vi "Data_Process_Mass.vi"(7 "Frequency Spectrum":cluster{sgl[], sgl[]}, 8 "error in":errorcluster, 9 "Mag. Frequency (kHz)":dbl format="%.5g", 10 "Cycl. Frequency (kHz)":dbl format="%.5g", 11 "Reference mass (u)":dbl format="%.5g") -> (0 "error out":errorcluster caption="sortie d'erreur", 3 "Mass Spectrum":cluster{"mass":sgl[], sgl[]})   [LabVIEW 2020]
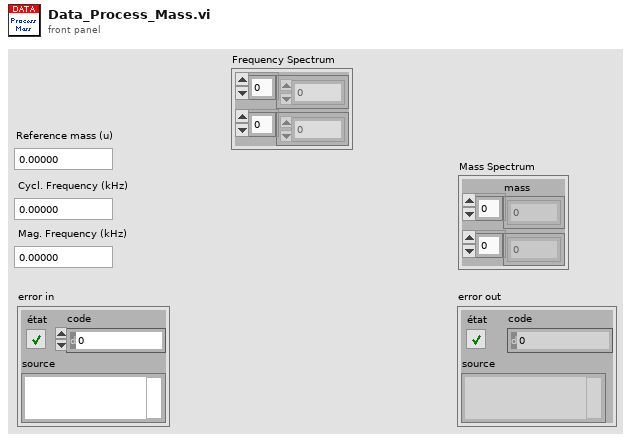
[diagram p1: front panel]
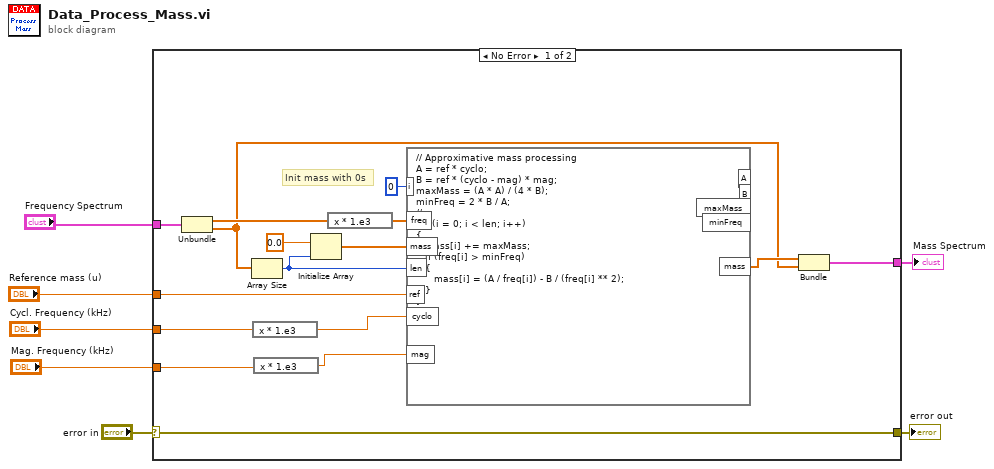
[diagram p0: block diagram]
diagram:
  n1 = case shown="No Error" "error in" {
    selector: "error in" -> [w23 w24]
    tunnel: [w23 w24] -> w6
    tunnel: "Frequency Spectrum" -> [w10 _]
    tunnel: "Reference mass (u)" -> [w20 _]
    tunnel: "Cycl. Frequency (kHz)" -> [w19 _]
    tunnel: "Mag. Frequency (kHz)" -> [w17 _]
    tunnel: [w13 _] -> w1
    frame No Error {
      # "Init mass with 0s"
      n2 = Unbundle(w10) -> (w9:sgl[], w8:sgl[])
      n3 = Array Size(array=w8) -> (size(s)=w15:i32)
      n4 = expression code="x * 1.e3"(w19) -> (w18:dbl)
      n5 = expression code="x * 1.e3"(w17) -> (w16:dbl)
      n6 = Initialize Array(sgl 0.0 ("élément"), w15) -> (w21:sgl[])
      n7 = expression code="x * 1.e3"(w9) -> (w12:sgl[])
      n8 = formula code="// Approximative mass processing\nA = ref * cyclo;\nB = ref * (cyclo - mag) * mag;\nmaxMass = (A * A) / (4 * B);\nminFreq = 2 * B / A;\n//\nfor (i = 0; i < len; i++)\n{\n   mass[i] += maxMass;\n   if (freq[i] > minFreq)\n   {\n      mass[i] = (A / freq[i]) - B / (freq[i] ** 2);\n   }\n}" ("Boîte de calcul")("freq"=w12, "mass"=w21, "ref"=w20, "cyclo"=w18, "mag"=w16, "len"=w15, "i"=0 ("variable en entrée")) -> ("mass"=w11:sgl[])  [unwired: 4 out]
      n9 = Bundle("mass"=w11, w8) -> (w13:cluster{"mass":sgl[], sgl[]})  [unwired: 1 in]
    }
    frame Error {
    }
  }
  "error out" <- w6
  "Mass Spectrum" <- w1
